vi "Constants.vi"() -> ()   [LabVIEW 2018]
panel:
  in  "HPMotionMagic":T1
  in  "HPIntakePositionPIDF":T2
  in  "4barPositionPIDF":T2
  in  "Gyro Angle \"Calibration\" Proportion":dbl
  in  "Drive Allowable Error":dbl=150.0
  in  "4bar horizantal position kF":dbl
  in  "4bar Encoder to Angle Ratio":dbl
  in  "Encoder Counts Per Rotation":dbl=4096.0
  in  "Wheel Diameter":dbl=6.0
  in  "HP Intake Wall":dbl
  in  "HP Intake Floor":dbl
  in  "HP Intake Home":dbl
  in  "RightDriveMotionMagic":T1
  in  "LeftDriveMotionMagic":T1
  in  "4bar Bottom Position":dbl
  in  "4bar Low Position":dbl
  in  "4bar Mid Position":dbl
  in  "4bar High Position":dbl
  in  "RightDrivePositionPIDF":T2
  in  "LeftDrivePositionPIDF":T2
  in  "Cargo Open Ramp":dbl=0.3
  in  "4bar Ramp":dbl=0.7
  in  "Drive Closed Loop Ramp":dbl=0.5
  in  "Drive Open Loop Ramp":dbl=0.5
  # "Intake STUFF"
  # "4bar STUFF"
  # "DRIVE STUFF"
  # "Make this F 0"
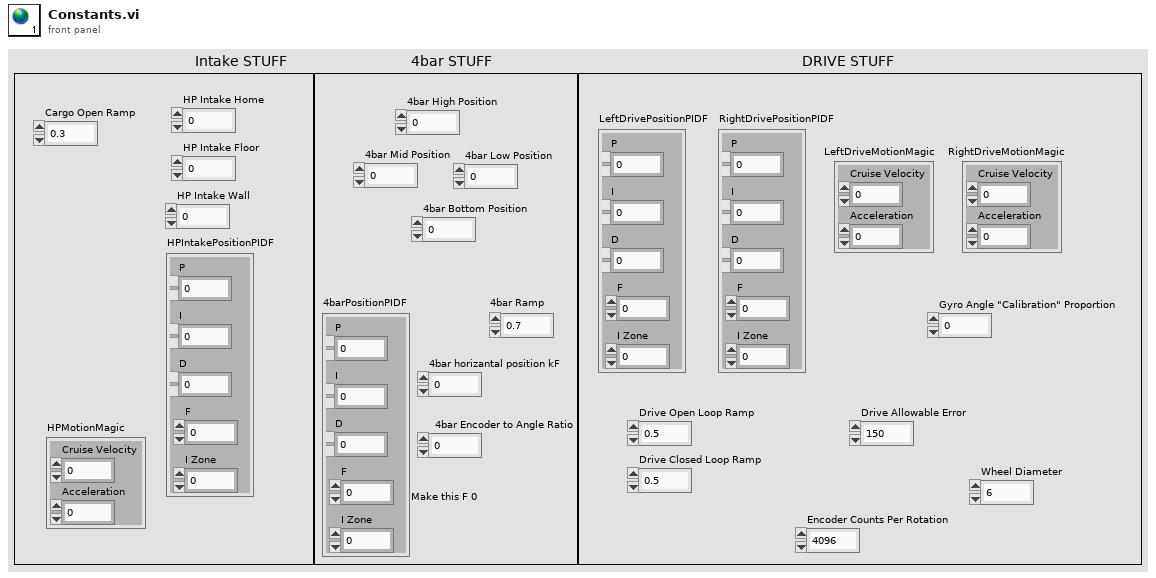
[diagram p1: front panel]
types:
  T1 = cluster{"Cruise Velocity":i32, "Acceleration":i32}
  T2 = cluster{"P":dbl, "I":dbl, "D":dbl, "F":dbl, "I Zone":dbl}
diagram:
